vi "Labview.vi"() -> ()   [LabVIEW 2020]
panel:
  out "Voltage":dbl(graph)
  out "Current":dbl(graph)
  in  "VISA resource name":refnum<visa-resource-name>
  in  "Table Control":string[][](table)
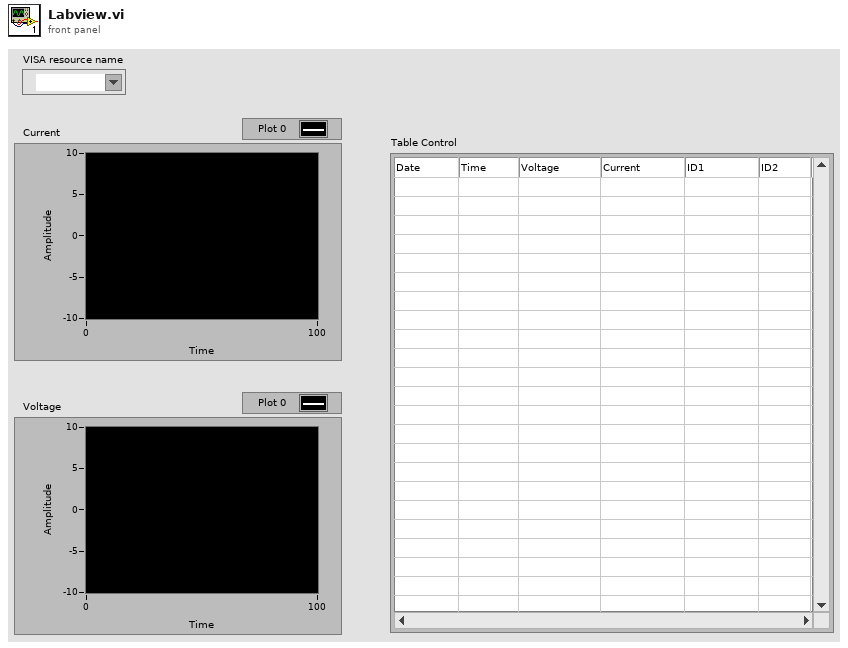
[diagram p1: front panel]
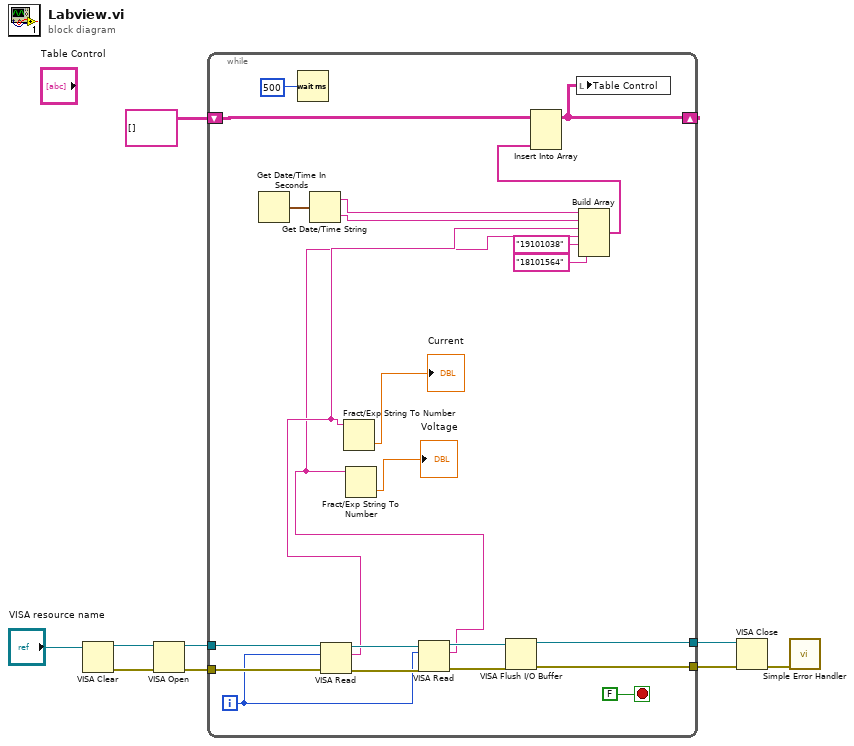
[diagram p0: block diagram]
diagram:
  n1 = VISA Clear(VISA resource name="VISA resource name") -> (VISA resource name out=w9:refnum<visa-resource-name>, error out=w8:errorcluster)  [unwired: 1 in]
  n2 = VISA Open(error in (no error)=w8, VISA resource name=w9) -> (VISA resource name=w6:refnum<visa-resource-name>, error out=w5:errorcluster)  [unwired: 3 in]
  n3 = while {
    tunnel: w6 -> [w32]
    tunnel: w5 -> [w31]
    tunnel: [w26] -> w4
    tunnel: [w25] -> w3
    shift-right: [w14] -> _
    shift-left: string[][] [] -> [w22]
    i -> [w24]
    stop <- FALSE stop-if-true
    n4 = Get Date/Time In Seconds() -> (seconds since 1Jan1904=w21:timestamp)
    n5 = Wait (ms)(milliseconds to wait=u32 500 ("millisecond timer value")) -> ()  [unwired: 1 out]
    n6 = Get Date/Time String(seconds (now)=w21) -> (date string=w20:string, time string=w19:string)  [unwired: 2 in]
    n7 = VISA Read(VISA resource name=w32, byte count=w24, error in (no error)=w31) -> (VISA resource name out=w30:refnum<visa-resource-name>, read buffer=w18:string, error out=w29:errorcluster)  [unwired: 1 out]
    n8 = Fract/Exp String To Number(string=w18) -> (number=→"Current":dbl)  [unwired: 3 in, 1 out]
    n9 = VISA Read(VISA resource name=w30, byte count=w24, error in (no error)=w29) -> (VISA resource name out=w28:refnum<visa-resource-name>, read buffer=w13:string, error out=w27:errorcluster)  [unwired: 1 out]
    n10 = Fract/Exp String To Number(string=w13) -> (number=→"Voltage":dbl)  [unwired: 3 in, 1 out]
    n11 = VISA Flush I/O Buffer(VISA resource name=w28, error in (no error)=w27) -> (VISA resource name out=w26:refnum<visa-resource-name>, error out=w25:errorcluster)  [unwired: 1 in]
    n12 = Build Array(w20, w19, w18, w13, "19101038" ("element"), "18101564" ("element")) -> (w17:string[])
    n13 = Insert Into Array(array=w22, new element=w17) -> (w14:string[][])  [unwired: 2 in]
    n14 = local write "Table Control"(w14) -> ()
  }
  n15 = VISA Close(VISA resource name=w4, error in (no error)=w3) -> (error out=w7:errorcluster)
  n16 = call <vilib>:"Simple Error Handler.vi"("error in (no error)"=w7) -> ()  [unwired: 4 in, 5 out]
